vi "Template Change Display Names for INI Import.vi"(8 "error in (no error)":errorcluster, 10 "Parameters":T2, 11 "Connection Refnum":T1) -> (0 "error out":errorcluster, 2 "Parameters 2":T2, 3 "Connection Refnum 2":T1)   [LabVIEW 2011]
uses:
  ITK EXT/utils/keyedarr.llb/Keyed Array.ctl
  Summitek EXT/ODBC/SQL Controls/Connection Refnum.ctl
  ITK EXT/utils/strutil.llb/Case Matching.ctl
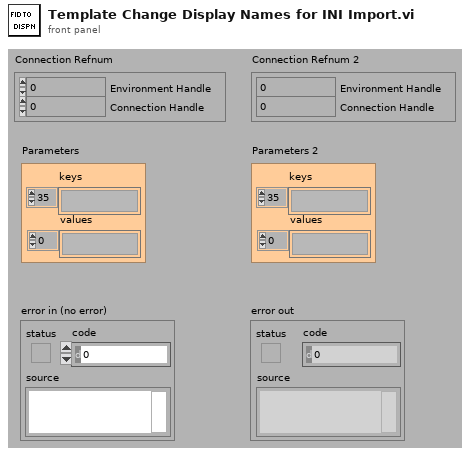
[diagram p1: front panel]
types:
  T1 = typedef "Connection Refnum.ctl" = cluster{"Environment Handle":i32, "Connection Handle":i32}
  T2 = typedef "Keyed Array.ctl" = cluster{"keys":string[], "values":string[]}
  T3 = typedef "Case Matching.ctl" = enum16{"a != A", "a == A", "system"}
  T4 = typedef "Field Record.ctl" = cluster{"ixField":i32, "iSequenceOrder":i32, "sxFieldId":string, "sxSequenceId":string, "sDisplayName":string, "sValue":string, "sUnits":string, "nDataType":T5, "nNextItem":T6, "fSystem":bool, "fSystemValue":bool, "fRequired":bool, "fSetAtTest":bool, "fTestField":bool, "fDeleted":bool, "fIndexed":bool, "fFreeList":bool}
  T5 = typedef "Field DataTypes.ctl" = enum32{"text", "numeric", "list", "timestamp", "boolean"}
  T6 = typedef "Field NextItem.ctl" = enum32{"Reset", "Retain", "Auto-Increment"}
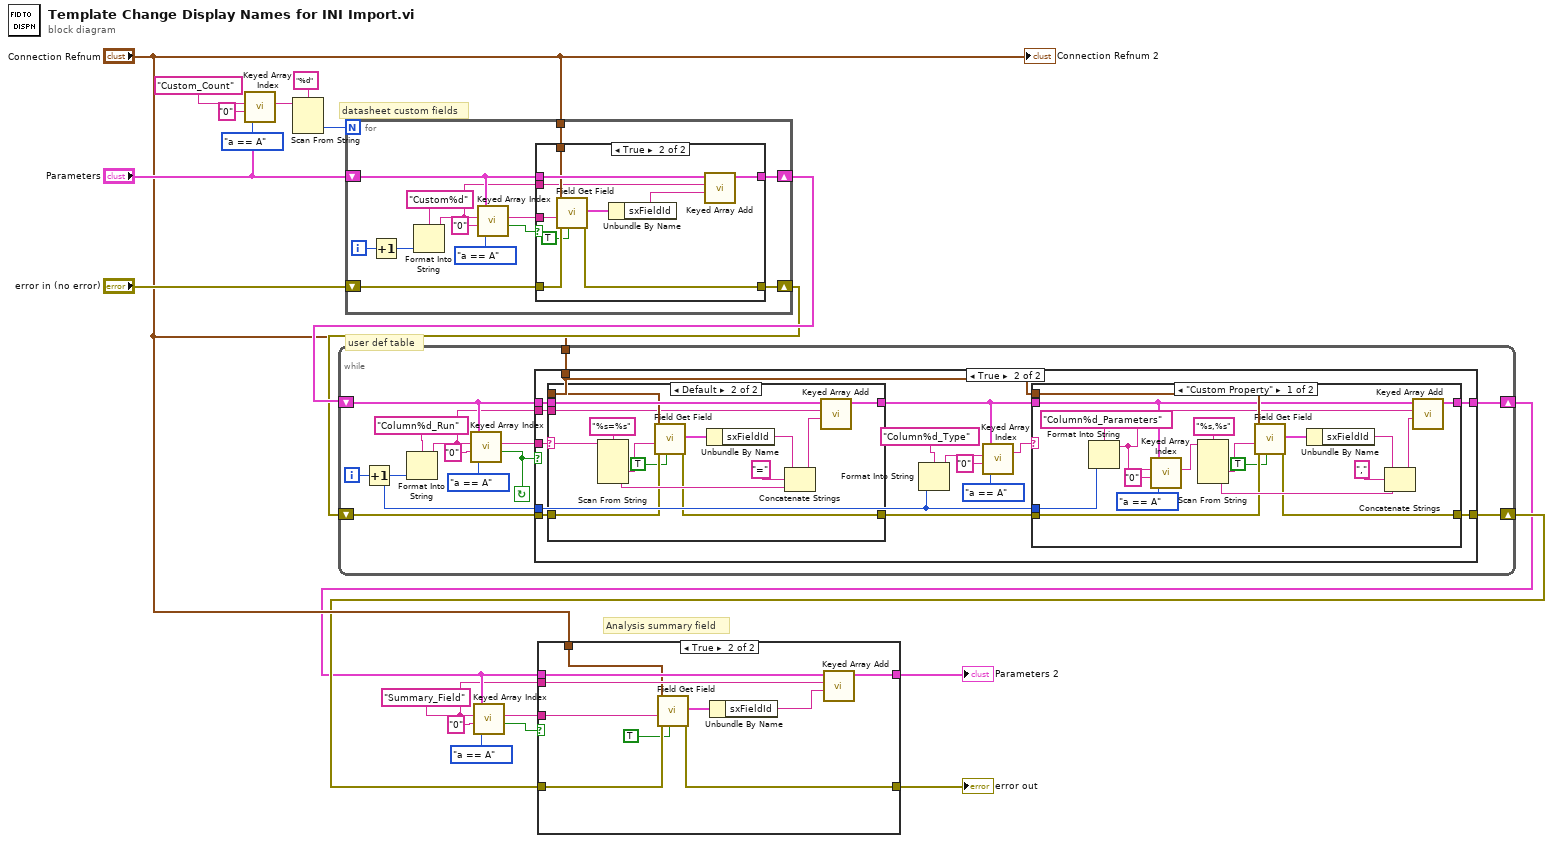
[diagram p0: block diagram]
diagram:
  w1 = "Summary_Field" ("key")
  # "Analysis summary field"
  # "user def table"
  # "datasheet custom fields"
  n1 = call "Keyed Array Index.vi"("case matching (sensitive)"=Case_Matching."a == A", "default value"="0", "key"="Custom_Count", "array in"="Parameters") -> ("value"=w16:string)  [unwired: 3 out]
  n2 = Scan From String(format string="%d", input string=w16) -> (output 1=w17:i32)  [unwired: 2 in, 4 out]
  n3 = for {
    N: w17 -> [_]
    tunnel: "Connection Refnum" -> [w27]
    shift-right: [w24] -> w11
    shift-left: "error in (no error)" -> [w25]
    shift-right: [w21] -> w12
    shift-left: "Parameters" -> [w28]
    i -> [w30]
    n4 = Increment(x=w30) -> (x+1=w29:i32)
    n5 = Format Into String(format string="Custom%d" ("key"), w29) -> (resulting string=w23:string)  [unwired: 2 in, 1 out]
    n6 = call "Keyed Array Index.vi"("case matching (sensitive)"=Case_Matching."a == A", "default value"="0", "key"=w23, "array in"=w28) -> ("valid key"=w22:bool, "value"=w26:string)  [unwired: 2 out]
    n7 = case shown="True" w22 {
      tunnel: w28 -> [w34 w45]
      tunnel: w27 -> [_ w44]
      tunnel: w26 -> [_ w43]
      tunnel: w25 -> [w35 w42]
      tunnel: [w35 w41] -> w24
      tunnel: w23 -> [_ w39]
      tunnel: [w34 w37] -> w21
      frame False {
      }
      frame True {
        n8 = call "Field Get Field.vi"("by sDisplayName? (f, by sFieldId)"=TRUE, "error in (no error)"=w42, "sFieldId or sDisplayName (\"\")"=w43, "Connection Refnum"=w44) -> ("error out"=w41:errorcluster, "Field"=w40:T4)  [unwired: 1 in, 5 out]
        n9 = Unbundle By Name(w40) -> ("sxFieldId"=w38:string)
        n10 = call "Keyed Array Add.vi"("value"=w38, "key"=w39, "array in"=w45) -> ("array out"=w37:T2)  [unwired: 1 in, 3 out]
      }
    }
  }
  n11 = while {
    tunnel: "Connection Refnum" -> [w53]
    shift-right: [w46] -> w9
    shift-left: w11 -> [w51]
    shift-right: [w49] -> w8
    shift-left: w12 -> [w54]
    i -> [w55]
    stop <- w48 continue-if-true
    n12 = Increment(x=w55) -> (x+1=w47:i32)
    n13 = Format Into String(format string="Column%d_Run" ("key"), w47) -> (resulting string=w50:string)  [unwired: 2 in, 1 out]
    n14 = call "Keyed Array Index.vi"("case matching (sensitive)"=Case_Matching."a == A", "default value"="0", "key"=w50, "array in"=w54) -> ("valid key"=w48:bool, "value"=w52:string)  [unwired: 2 out]
    n15 = case shown="True" w48 {
      tunnel: w54 -> [w60 w75]
      tunnel: w53 -> [_ w64]
      tunnel: w52 -> [_ w73]
      tunnel: w51 -> [w59 w69]
      tunnel: w50 -> [_ w74]
      tunnel: [w60 w66] -> w49
      tunnel: w47 -> [_ w62]
      tunnel: [w59 w65] -> w46
      frame False {
      }
      frame True {
        n16 = case shown="Default" w73 {
          selector: w73 -> [_ w108]
          tunnel: w75 -> [w98 w113]
          tunnel: w64 -> [_ w112]
          tunnel: w74 -> [_ w110]
          tunnel: [w98 w109] -> w67
          tunnel: w69 -> [w97 w101]
          tunnel: [w97 w100] -> w68
          frame "most recent" {
          }
          frame Default {
            n17 = Scan From String(format string="%s=%s", input string=w108) -> (output 1=w106:string, output 2=w103:string)  [unwired: 2 in, 5 out]
            n18 = call "Field Get Field.vi"("by sDisplayName? (f, by sFieldId)"=TRUE, "error in (no error)"=w101, "sFieldId or sDisplayName (\"\")"=w106, "Connection Refnum"=w112) -> ("error out"=w100:errorcluster, "Field"=w111:T4)  [unwired: 1 in, 5 out]
            n19 = Unbundle By Name(w111) -> ("sxFieldId"=w105:string)
            n20 = Concatenate Strings(w105, "=" ("format string"), w103) -> (w104:string)
            n21 = call "Keyed Array Add.vi"("value"=w104, "key"=w110, "array in"=w113) -> ("array out"=w109:T2)  [unwired: 1 in, 3 out]
          }
        }
        n22 = Format Into String(format string="Column%d_Type" ("key"), w62) -> (resulting string=w72:string)  [unwired: 2 in, 1 out]
        n23 = call "Keyed Array Index.vi"("case matching (sensitive)"=Case_Matching."a == A", "default value"="0", "key"=w72, "array in"=w67) -> ("value"=w63:string)  [unwired: 3 out]
        n24 = case shown="\"Custom Property\"" w63 {
          tunnel: w67 -> [w80 w96]
          tunnel: w64 -> [w94 _]
          tunnel: [w92 w96] -> w66
          tunnel: w68 -> [w85 w95]
          tunnel: [w84 w95] -> w65
          tunnel: w62 -> [w82 _]
          frame "Custom Property" {
            n25 = Format Into String(format string="Column%d_Parameters" ("key"), w82) -> (resulting string=w77:string)  [unwired: 2 in, 1 out]
            n26 = call "Keyed Array Index.vi"("case matching (sensitive)"=Case_Matching."a == A", "default value"="0", "key"=w77, "array in"=w80) -> ("value"=w79:string)  [unwired: 3 out]
            n27 = Scan From String(format string="%s,%s", input string=w79) -> (output 1=w90:string, output 2=w87:string)  [unwired: 2 in, 5 out]
            n28 = call "Field Get Field.vi"("by sDisplayName? (f, by sFieldId)"=TRUE, "error in (no error)"=w85, "sFieldId or sDisplayName (\"\")"=w90, "Connection Refnum"=w94) -> ("error out"=w84:errorcluster, "Field"=w93:T4)  [unwired: 1 in, 5 out]
            n29 = Unbundle By Name(w93) -> ("sxFieldId"=w89:string)
            n30 = Concatenate Strings(w89, "," ("format string"), w87) -> (w88:string)
            n31 = call "Keyed Array Add.vi"("value"=w88, "key"=w77, "array in"=w80) -> ("array out"=w92:T2)  [unwired: 1 in, 3 out]
          }
          frame Default {
          }
        }
      }
    }
  }
  n32 = call "Keyed Array Index.vi"("case matching (sensitive)"=Case_Matching."a == A", "default value"="0", "key"=w1, "array in"=w8) -> ("valid key"=w4:bool, "value"=w5:string)  [unwired: 2 out]
  n33 = case shown="True" w4 {
    tunnel: w8 -> [w115 w125]
    tunnel: "Connection Refnum" -> [_ w122]
    tunnel: w5 -> [_ w120]
    tunnel: w9 -> [w114 w123]
    tunnel: w1 -> [_ w124]
    tunnel: [w115 w117] -> w3
    tunnel: [w114 w118] -> w2
    frame False {
    }
    frame True {
      n34 = call "Field Get Field.vi"("by sDisplayName? (f, by sFieldId)"=TRUE, "error in (no error)"=w123, "sFieldId or sDisplayName (\"\")"=w120, "Connection Refnum"=w122) -> ("error out"=w118:errorcluster, "Field"=w121:T4)  [unwired: 1 in, 5 out]
      n35 = Unbundle By Name(w121) -> ("sxFieldId"=w119:string)
      n36 = call "Keyed Array Add.vi"("value"=w119, "key"=w124, "array in"=w125) -> ("array out"=w117:T2)  [unwired: 1 in, 3 out]
    }
  }
  "Parameters 2" <- w3
  "error out" <- w2
  "Connection Refnum 2" <- "Connection Refnum"
